vi "Escape-Unescape String for XML.vi"(9 "attribute? (F: entity)":bool, 10 "String":string, 11 "Action (Escape)":enum16{"Escape", "Unescape"}(ring)) -> (2 "String out":string)   [LabVIEW 2013]
panel:
  # "Copyright © 2006-2008 James Kring, Inc. All rights reserved.\n\nAuthor: Jim Kring <jim.kring@jameskring.com>\n\nThis library is provided \"AS IS\" , WITHOUT WARRANTIES OR \nCONDITIONS OF ANY KIND, either express or implied.\n\nJames Kring, Inc. -- http://www.jameskring.com"
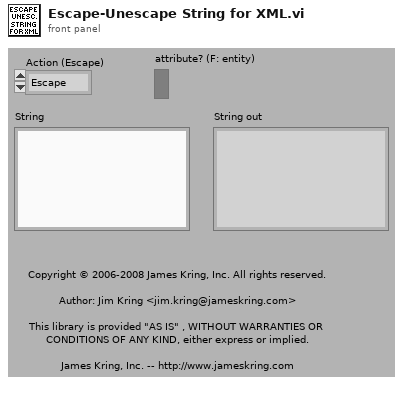
[diagram p1: front panel]
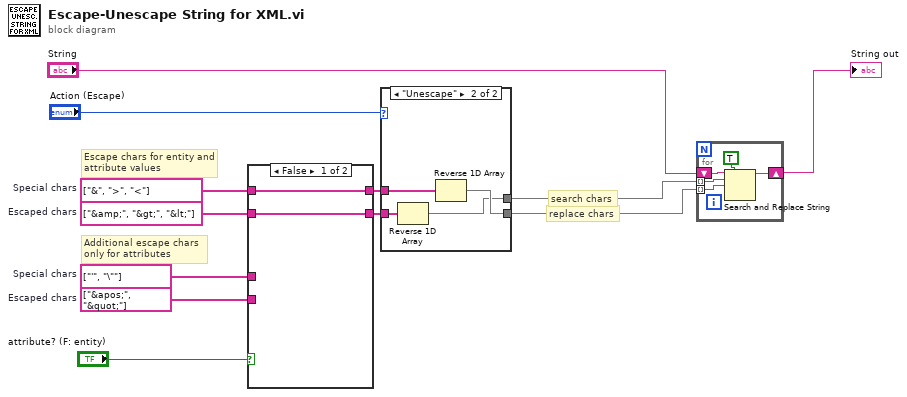
[diagram p0: block diagram]
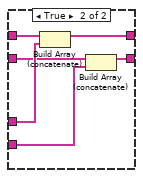
[diagram p2: hidden frame]
diagram:
  w5 = string[] ["&apos;", "&quot;"]  # Escaped chars
  w6 = string[] ["'", "\""]  # Special chars
  w8 = string[] ["&amp;", "&gt;", "&lt;"]  # Escaped chars
  w10 = string[] ["&", ">", "<"]  # Special chars
  # "replace chars"
  # "search chars"
  # "Escape chars for entity and attribute values"
  # "Additional escape chars only for attributes"
  n1 = case shown="False" "attribute? (F: entity)" {
    tunnel: [w14 w16] -> w9
    tunnel: w10 -> [w14 w20]
    tunnel: [w13 w17] -> w7
    tunnel: w8 -> [w13 w18]
    tunnel: w6 -> [_ w19]
    tunnel: w5 -> [_ w15]
    frame False {
    }
    frame True {
      n2 = Build Array (concatenate)(w20, w19) -> (w16:string[])
      n3 = Build Array (concatenate)(w18, w15) -> (w17:string[])
    }
  }
  n4 = case shown="\"Unescape\"" "Action (Escape)" {
    tunnel: w9 -> [w22 w26]
    tunnel: w7 -> [w21 w24]
    tunnel: [w22 w23] -> w4
    tunnel: [w21 w25] -> w3
    frame "Escape" {
    }
    frame "Unescape" {
      n5 = Reverse 1D Array(array=w24) -> (reversed array=w23:string[])
      n6 = Reverse 1D Array(array=w26) -> (reversed array=w25:string[])
    }
  }
  n7 = for {
    tunnel: w4 -> [w31] mode=indexing
    tunnel: w3 -> [w30] mode=indexing
    shift-right: [w28] -> w1
    shift-left: "String" -> [w27]
    n8 = Search and Replace String(replace all?=TRUE ("replace all? (F)"), input string=w27, search string=w31, replace string=w30) -> (result string=w28:string)  [unwired: 4 in, 3 out]
  }
  "String out" <- w1
